vi "lotterygen.vi"() -> ()   [LabVIEW 2019]
panel:
  out "lucky number":dbl
  out "s? t:f":string
  out "Array":string[](array[string])
  out "sum":i32
  in  "String":string
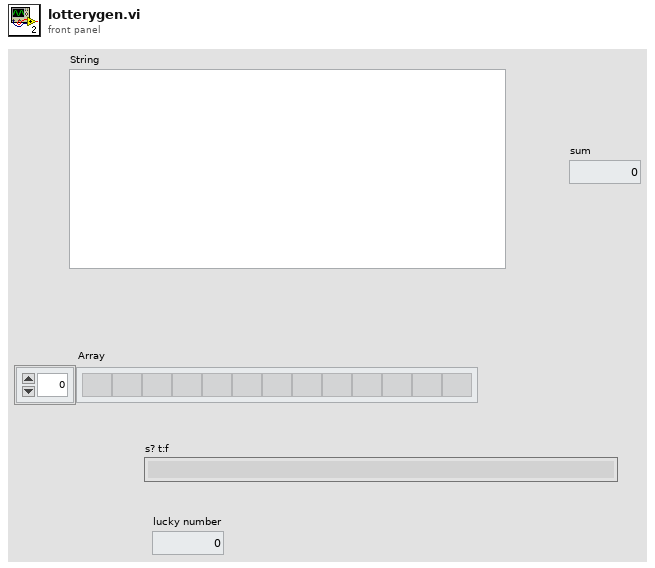
[diagram p1: front panel]
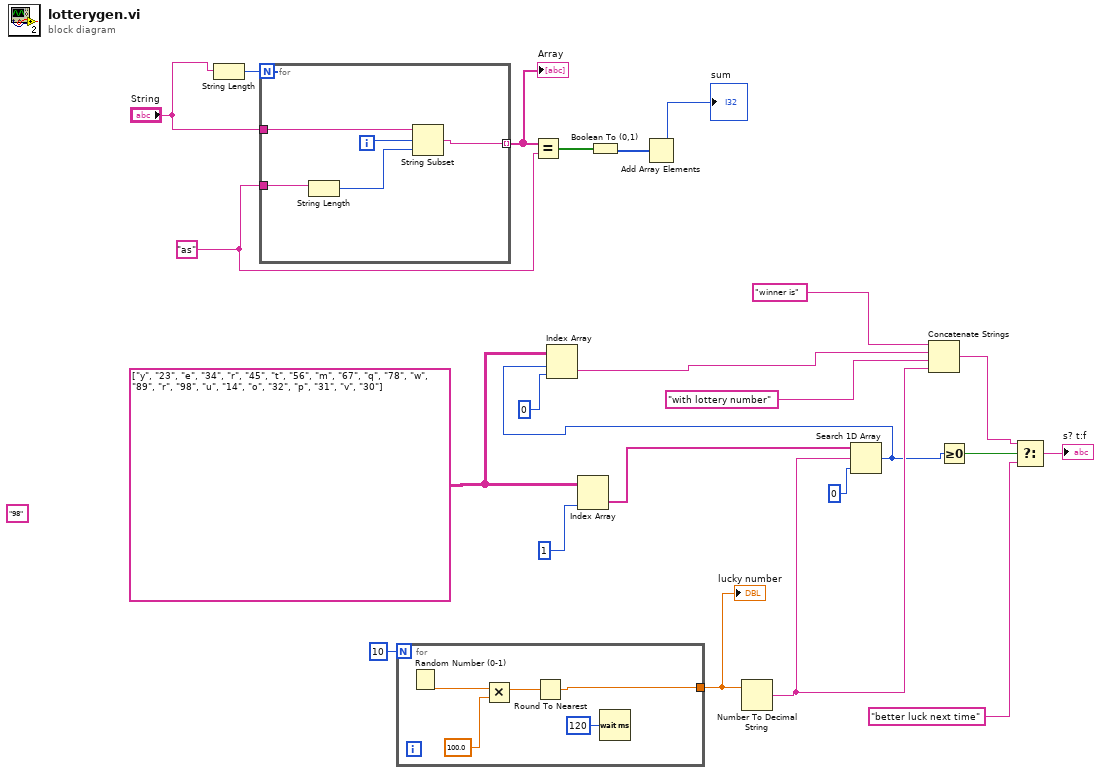
[diagram p0: block diagram]
diagram:
  (unwired) "98"
  w12 = string[][] [["y", "23"], ["e", "34"], ["r", "45"], ["t", "56"], ["m", "67"], ["q", "78"], ["w", "89"], ["r", "98"], ["u", "14"], ["o", "32"], ["p", "31"], ["v", "30"]]
  w21 = "as"
  n1 = String Length(string="String") -> (length=w23:i32)
  n2 = for {
    N: w23 -> [_]
    tunnel: "String" -> [w28]
    tunnel: w21 -> [w26]
    tunnel: [w24] -> w17 mode=indexing
    i -> [w27]
    n3 = String Length(string=w26) -> (length=w25:i32)
    n4 = String Subset(string=w28, offset (0)=w27, length (rest)=w25) -> (substring=w24:string)
  }
  "Array" <- w17
  n5 = for {
    N: 10 -> [_]
    tunnel: [w31] -> w2
    n6 = Random Number (0-1)() -> (number: 0 to 1=w33:dbl)
    n7 = Multiply(x=w33, y=100.0) -> (x*y=w32:dbl)
    n8 = Round To Nearest(number=w32) -> (nearest integer value=w31:dbl)
    n9 = Wait (ms)(milliseconds to wait=u32 120) -> ()  [unwired: 1 out]
  }
  "lucky number" <- w2
  n10 = Equal?(x=w17, y=w21) -> (x = y?=w20:bool[])
  n11 = Index Array "Index Array"(array=w12, index (col)=1 ("disabled index (col)")) -> (element=w14:string[])  [unwired: 1 in]
  n12 = Boolean To (0,1)(Boolean=w20) -> (0, 1=w19:i16[])
  n13 = Add Array Elements(numeric array=w19) -> (sum=→"sum":i16)
  n14 = Number To Decimal String(number=w2) -> (decimal integer string=w7:string)  [unwired: 1 in]
  n15 = Search 1D Array(1D array=w14, element=w7, start index (0)=0) -> (index of element=w1:i32)
  n16 = Index Array(array=w12, index (row)=w1, index (col)=0 ("disabled index (col)")) -> (element=w9:string)
  n17 = Concatenate Strings("winner is" ("string"), w9, "with lottery number" ("string"), w7) -> (w5:string)
  n18 = Greater Or Equal To 0?(x=w1) -> (x >= 0?=w6:bool)
  n19 = Select(t=w5, s=w6, f="better luck next time") -> (s? t:f=→"s? t:f":string)
